vi "driver enable and absolute move.vi"(8 "error in (no error)":errorcluster, 9 "Numeric in":dbl, 10 "Numeric 3":i32, 11 "ZaberASeries in":refnum<class "ZaberASeries.lvclass">) -> (0 "error out":errorcluster, 2 "time to move (ms)":dbl, 3 "ZaberASeries out":refnum<class "ZaberASeries.lvclass">)   [LabVIEW 2020, in "ZaberASeries.lvclass"]
uses:
  ZaberASeries.lvclass
  OnOffTypeDef.ctl
  ZaberASeries.lvclass/ZaberASeries.ctl
  Zaber A Series.lvlib
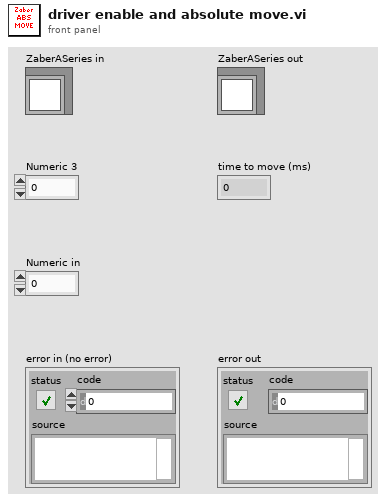
[diagram p1: front panel]
types:
  T1 = typedef "OnOffTypeDef.ctl" = enum16{"off", "on"}
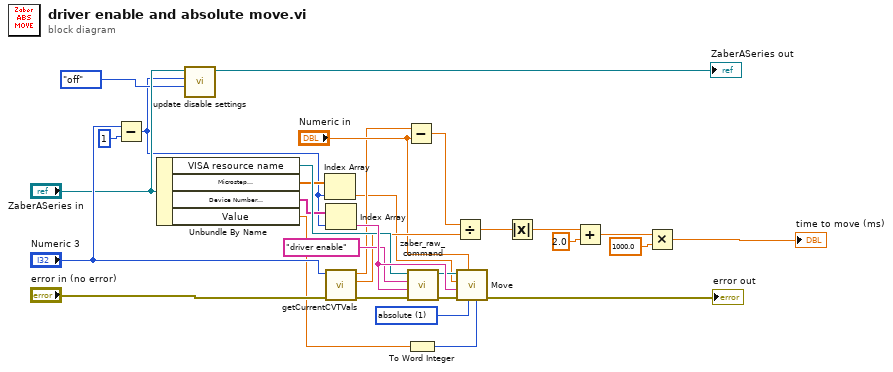
[diagram p0: block diagram]
diagram:
  w9 = u16 1 items=["relative", "absolute"] ("Movement Type (0: relative)")
  n1 = Subtract(x="Numeric 3", y=1) -> (x-y=w1:i32)
  n2 = Unbundle By Name("ZaberASeries in") -> ("VISA resource name"=w22:refnum<visa-resource-name>, "Microstep\nSizes"=w5:dbl[], "Device Number\n& Axis"=w6:string[], "Value"=w7:dbl)
  n3 = call-dynamic "update disable settings.vi"("disable"=OnOffTypeDef."off" ("new element/subarray"), "channel index"=w1, "ZaberASeries in"="ZaberASeries in") -> ("ZaberASeries out"=→"ZaberASeries out":refnum<class "ZaberASeries.lvclass">)  [unwired: 8 in]
  n4 = Index Array(array=w5, index=w1) -> (element=w10:dbl)
  n5 = Index Array(array=w6, index=w1) -> (element=w30:string)
  n6 = call "getCurrentCVTVals.vi"("error in"="error in (no error)", "channel number"="Numeric 3") -> ("error out"=w20:errorcluster, "speed"=w17:dbl, "position"=w14:dbl)  [unwired: 7 in]
  n7 = Subtract(x=w14, y="Numeric in") -> (x-y=w16:dbl)
  n8 = To Word Integer(number=w7) -> (16bit integer=w8:i16)
  n9 = call "zaber_raw_command.vi"("error in (no error)"=w20, "Device and Axis"=w30, "Command"="driver enable", "VISA Refnum in"=w22) -> ("error out"=w21:errorcluster, "VISA resource name out"=w23:refnum<visa-resource-name>)  [unwired: 2 in, 4 out]
  n10 = Divide(x=w16, y=w17) -> (x/y=w18:dbl)
  n11 = call "Move.vi"("Units (0: microsteps)"=w8, "Movement Type (0: relative)"=w9, "Move Distance (0)"="Numeric in", "error in (no error)"=w21, "Device and Axis"=w30, "Microstep Size (0)"=w10, "VISA resource name"=w23) -> ("error out"=→"error out":errorcluster)  [unwired: 3 in, 1 out]
  n12 = Absolute Value(x=w18) -> (abs(x)=w27:dbl)
  n13 = Add(x=w27, y=2.0) -> (x+y=w28:dbl)
  n14 = Multiply(x=w28, y=1000.0) -> (x*y=→"time to move (ms)":dbl)
